vi "Decimation - time to write.vi"(10 "Iteration":i32, 11 "Decimation":u32) -> (3 "Ready":bool)   [LabVIEW 2013, in "RefMem DMA Custom Device.lvlib"]
uses:
  RefMem DMA Custom Device.lvlib
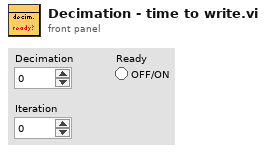
[diagram p1: front panel]
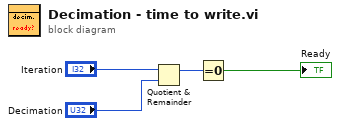
[diagram p0: block diagram]
diagram:
  n1 = Quotient & Remainder(x="Iteration", y="Decimation") -> (x-y*floor(x/y)=w2:u32)  [unwired: 1 out]
  n2 = Equal To 0?(x=w2) -> (x = 0?=→"Ready":bool)
